vi "Cyclic_Synchronous_Position_Mode.vi"() -> ()   [LabVIEW 2014]
uses:
  <vilib>/Motion/plugins/Delta SDI Plug-in/Delta Support Files/Test VIs/SDI Status PDOs.ctl
panel:
  out "Status Word":u16(graph)
  out "SDI Status PDOs":T1
  in  "stop":bool
  in  "1st RxPDO Mapping-TargetPosition":i32
  out "error out":errorcluster
  # "6060h:\n\n0: Reserved\n1: Profile Position Mode\n3: Profile Velocity Mode\n4: Profile Torque Mode\n6: Homing Mode\n7: Interpolated Position Mode\n8: Cyclic Synchronous Position Mode\n9: Cyclic Synchronous Velocity Mode\n10: Cyclic Synchronous Torque Mode"
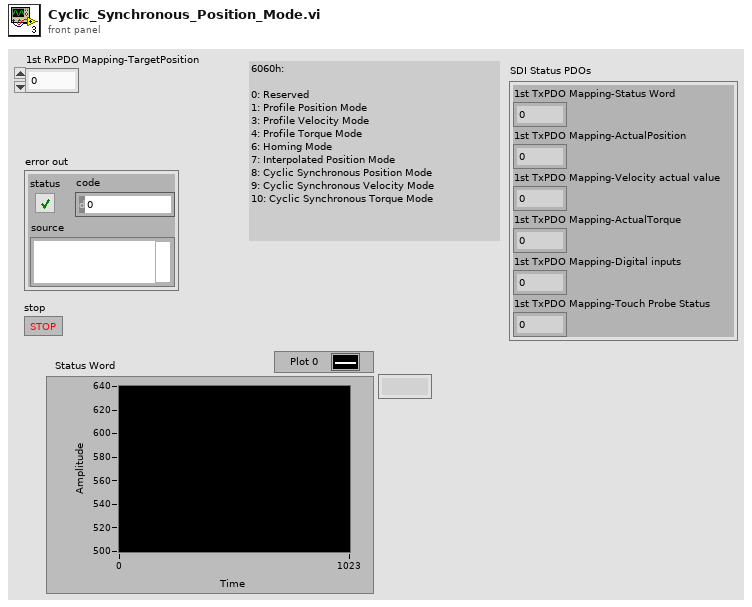
[diagram p1: front panel]
types:
  T1 = typedef "SDI Status PDOs.ctl" = cluster{"1st TxPDO Mapping-Status Word":u16, "1st TxPDO Mapping-ActualPosition":i32, "1st TxPDO Mapping-Velocity actual value":i32, "1st TxPDO Mapping-ActualTorque":i16, "1st TxPDO Mapping-Digital inputs":u32, "1st TxPDO Mapping-Touch Probe Status":u16}
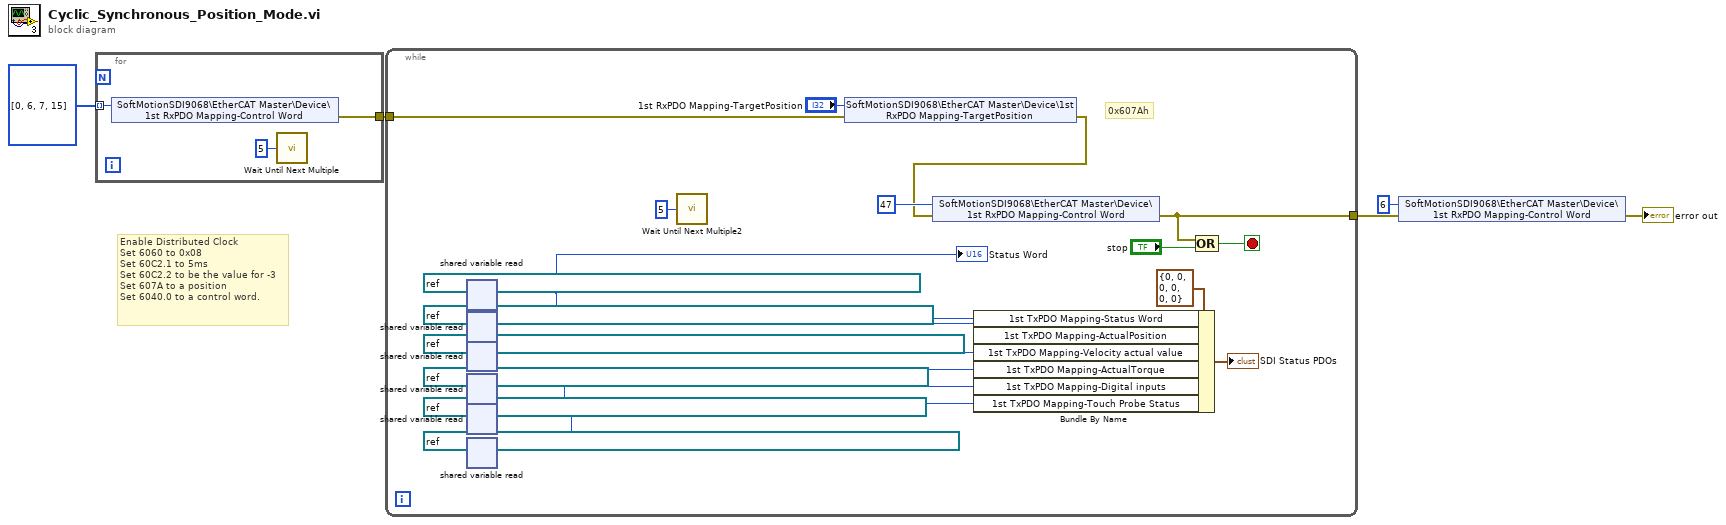
[diagram p0: block diagram]
diagram:
  # "Enable Distributed Clock\nSet 6060 to 0x08\nSet 60C2.1 to 5ms\nSet 60C2.2 to be the value for -3\nSet 607A to a position\nSet 6040.0 to a control word."
  n1 = for {
    tunnel: u16[] [0, 6, 7, 15] -> [w8] mode=indexing
    tunnel: [w6] -> w2
    n2 = shared-variable "SoftMotionSDI9068\\EtherCAT Master\\Device\\1st RxPDO Mapping-Control Word"(w8) -> (error out=w6:errorcluster)  [unwired: 1 in]
    n3 = call "Wait Until Next Multiple"("Count(mSec)"=u32 5) -> ()  [unwired: 1 out]
  }
  n4 = while {
    tunnel: w2 -> [w26]
    tunnel: [w24] -> w1
    stop <- w25 stop-if-true
    # "0x607Ah"
    n5 = shared-variable-read(refnum<k21> "ni.var.io://SoftMotionSDI9068/EtherCAT Master/Device/1st TxPDO Mapping-Status Word" ("shared variable refnum in")) -> (w15:u16)  [unwired: 1 in, 2 out]
    "Status Word" <- w15
    n6 = shared-variable-read(refnum<k21> "ni.var.io://SoftMotionSDI9068/EtherCAT Master/Device/1st TxPDO Mapping-ActualPosition" ("shared variable refnum in")) -> (w18:i32)  [unwired: 1 in, 2 out]
    n7 = shared-variable-read(refnum<k21> "ni.var.io://SoftMotionSDI9068/EtherCAT Master/Device/1st TxPDO Mapping-Velocity actual value" ("shared variable refnum in")) -> (w19:i32)  [unwired: 1 in, 2 out]
    n8 = shared-variable-read(refnum<k21> "ni.var.io://SoftMotionSDI9068/EtherCAT Master/Device/1st TxPDO Mapping-ActualTorque" ("shared variable refnum in")) -> (w20:i16)  [unwired: 1 in, 2 out]
    n9 = shared-variable-read(refnum<k21> "ni.var.io://SoftMotionSDI9068/EtherCAT Master/Device/1st TxPDO Mapping-Digital inputs" ("shared variable refnum in")) -> (w21:u32)  [unwired: 1 in, 2 out]
    n10 = shared-variable-read(refnum<k21> "ni.var.io://SoftMotionSDI9068/EtherCAT Master/Device/1st TxPDO Mapping-Touch Probe Status" ("shared variable refnum in")) -> (w22:u16)  [unwired: 1 in, 2 out]
    n11 = call "Wait Until Next Multiple2"("Count(mSec)"=u32 5) -> ()  [unwired: 1 out]
    n12 = shared-variable "SoftMotionSDI9068\\EtherCAT Master\\Device\\1st RxPDO Mapping-TargetPosition"("1st RxPDO Mapping-TargetPosition", error in=w26) -> (error out=w23:errorcluster)
    n13 = shared-variable "SoftMotionSDI9068\\EtherCAT Master\\Device\\1st RxPDO Mapping-Control Word"(u16 47 ("1st RxPDO Mapping-Control Word"), error in=w23) -> (error out=w24:errorcluster)
    n14 = Bundle By Name(cluster=T1 {"1st TxPDO Mapping-Status Word"=0, "1st TxPDO Mapping-ActualPosition"=0, "1st TxPDO Mapping-Velocity actual value"=0, "1st TxPDO Mapping-ActualTorque"=0, "1st TxPDO Mapping-Digital inputs"=0, "1st TxPDO Mapping-Touch Probe Status"=0} ("SDI Status PDOs"), "1st TxPDO Mapping-Status Word"=w15, "1st TxPDO Mapping-ActualPosition"=w18, "1st TxPDO Mapping-Velocity actual value"=w19, "1st TxPDO Mapping-ActualTorque"=w20, "1st TxPDO Mapping-Digital inputs"=w21, "1st TxPDO Mapping-Touch Probe Status"=w22) -> (→"SDI Status PDOs":T1)
    n15 = Compound Arithmetic op=OR(w24, "stop") -> (w25:bool)
  }
  n16 = shared-variable "SoftMotionSDI9068\\EtherCAT Master\\Device\\1st RxPDO Mapping-Control Word"(u16 6 ("1st RxPDO Mapping-Control Word"), error in=w1) -> (error out=→"error out":errorcluster)
